vi "XML Reader Start Root.vi"(8 "error in":errorcluster, 10 "Root Name":string="Calibration", 11 "XML Reader In":T1) -> (0 "error out":errorcluster, 3 "XML Reader Out":T1)   [LabVIEW 2016, in "Pathloss XML Reader.lvlib"]
uses:
  Pathloss XML Reader.lvlib
  Controls/XML Reader Data Ref.ctl
  Controls/XML Reader Data.ctl
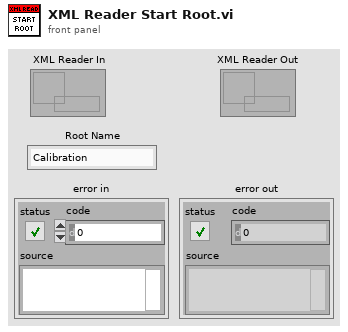
[diagram p1: front panel]
types:
  T1 = typedef "Pathloss XML Reader.lvlib/XML Reader Data Ref.ctl" = refnum<data-value>
  T2 = typedef "Pathloss XML Reader.lvlib/XML Reader Data.ctl" = cluster{"Remaining XML":string, "Section Name Stack":string[], "Section Stack":string[]}
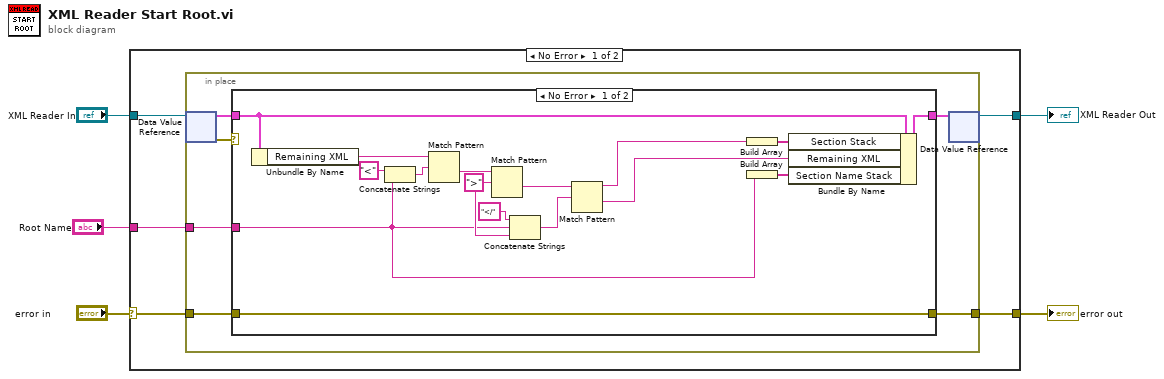
[diagram p0: block diagram]
diagram:
  n1 = case shown="No Error" "error in" {
    selector: "error in" -> [w8 w35]
    tunnel: [w7 w35] -> w5
    tunnel: [w9 w36] -> w4
    tunnel: "XML Reader In" -> [w10 w36]
    tunnel: "Root Name" -> [w6 _]
    frame No Error {
      n2 = in-place {
        in-place-border: w8 -> [w13]
        in-place-border: [w12] -> w7
        in-place-border: w6 -> [w11]
        n3 = in-place-dvr #1(w10) -> (w15:T2, w16:errorcluster)
        n4 = case shown="No Error" w16 {
          selector: w16 -> [_ w33]
          tunnel: w15 -> [w32 w34]
          tunnel: [w31 w34] -> w14
          tunnel: w13 -> [w27 _]
          tunnel: [w27 w33] -> w12
          tunnel: w11 -> [w22 _]
          frame No Error {
            w26 = ">" ("regular expression")
            n5 = Unbundle By Name(w32) -> ("Remaining XML"=w24:string)
            n6 = Concatenate Strings("<" ("string"), w22) -> (w29:string)
            n7 = Match Pattern(string=w24, regular expression=w29) -> (after substring=w28:string)  [unwired: 1 in, 3 out]
            n8 = Match Pattern(string=w28, regular expression=w26) -> (after substring=w20:string)  [unwired: 1 in, 3 out]
            n9 = Concatenate Strings("</" ("string"), w22, w26) -> (w19:string)
            n10 = Match Pattern(string=w20, regular expression=w19) -> (before substring=w18:string, after substring=w17:string)  [unwired: 1 in, 2 out]
            n11 = Build Array(w18) -> (w21:string[])
            n12 = Build Array(w22) -> (w23:string[])
            n13 = Bundle By Name(cluster=w32, "Section Stack"=w21, "Remaining XML"=w17, "Section Name Stack"=w23) -> (w31:T2)
          }
          frame Error {
          }
        }
        n14 = in-place-dvr #1(w14) -> (w9:T1)  [unwired: 1 out]
      }
    }
    frame Error {
    }
  }
  "error out" <- w5
  "XML Reader Out" <- w4
